vi "Set Power.vi"(8 "error in (no error)":errorcluster, 9 "Right Power":dbl min=-1.0 max=1.0, 10 "Left Power":dbl min=-1.0 max=1.0, 11 "Logical Forward Drive in":refnum<class "Forward Drive.lvclass">) -> (0 "error out":errorcluster, 3 "Logical Forward Drive out":refnum<class "Forward Drive.lvclass">)   [LabVIEW 2014, in "Forward Drive.lvlib" / "Forward Drive.lvclass"]
uses:
  Forward Drive.lvclass
  Motor with Encoders/Motors with Encoders Messages/Set Rate (Percent) Msg/Set Rate (Percent) Msg.lvclass/Set Rate (Percent) Msg.ctl
  <vilib>/ActorFramework/Message Enqueuer/Message Enqueuer.lvclass/Message Enqueuer.ctl
  <vilib>/ActorFramework/Message Enqueuer/Enqueue.vi
  <vilib>/ActorFramework/Message Priority Queue/Priority Enqueue.vi
  Motor with Encoders/Motors with Encoders Messages/Set Rate (Percent) Msg/Set Rate (Percent) Msg.lvclass
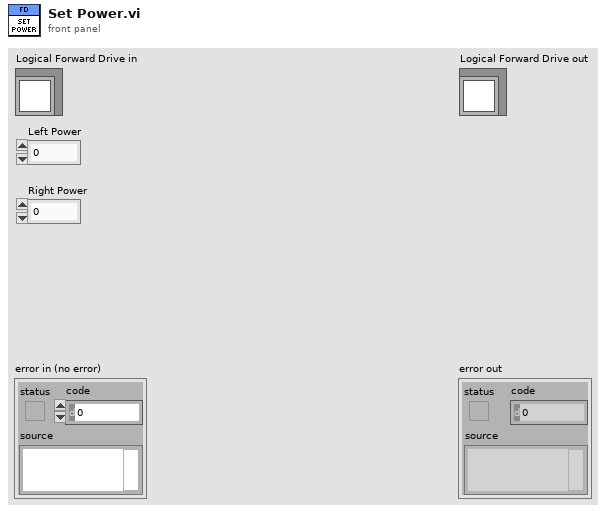
[diagram p1: front panel]
types:
  T1 = enum16{"Critical", "Error", "Warning", "Informational", "Debug"}
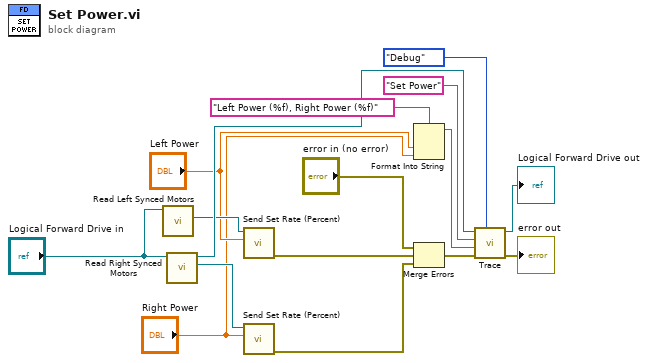
[diagram p0: block diagram]
diagram:
  n1 = call-dynamic "Read Left Synced Motors.vi"("Forward Drive in"="Logical Forward Drive in") -> ("Actor Framework:Message Enqueuer"=w6:refnum<class "Message Enqueuer.lvclass">)  [unwired: 8 in, 2 out]
  n2 = call-dynamic "Read Right Synced Motors.vi"("Forward Drive in"="Logical Forward Drive in") -> ("Actor Framework:Message Enqueuer"=w4:refnum<class "Message Enqueuer.lvclass">, "Forward Drive out"=w15:refnum<class "Forward Drive.lvclass">)  [unwired: 8 in, 1 out]
  n3 = call "Send Set Rate (Percent).vi"("Rate (Percentage)"="Left Power", "Message Enqueuer"=w6) -> ("error out"=w2:errorcluster)  [unwired: 8 in, 1 out]
  n4 = call "Send Set Rate (Percent).vi"("Rate (Percentage)"="Right Power", "Message Enqueuer"=w4) -> ("error out"=w1:errorcluster)  [unwired: 8 in, 1 out]
  n5 = Format Into String(format string="Left Power (%f), Right Power (%f)", "Left Power", "Right Power") -> (resulting string=w10:string)  [unwired: 2 in, 1 out]
  n6 = Merge Errors("error in (no error)", w2, w1) -> (w7:errorcluster)
  n7 = call-dynamic "Trace.vi"("Trace Level"=T1."Debug", "error in (no error)"=w7, "System Message"=w10, "System Action"="Set Power" ("System Message"), "System Actor in"=w15) -> ("error out"=→"error out":errorcluster, "System Actor out"=→"Logical Forward Drive out":refnum<class "Forward Drive.lvclass">)  [unwired: 5 in]
